vi "Homework-8 previous next Correct.vi"() -> ()   [LabVIEW 2016]
uses:
  <vilib>/Utility/file.llb/Read Delimited Spreadsheet (DBL).vi
panel:
  out "file name":string
  in  "stop":bool
  out "Waveform Graph":dbl[](graph)
  out "first row":dbl[](array[numeric])
  out "filenames":string[](array[string])
  out "folder names":string[](array[string])
  out "stripped path":path
  out "selected path":path
  out "File path":path
  in  "next":bool
  in  "previous":bool
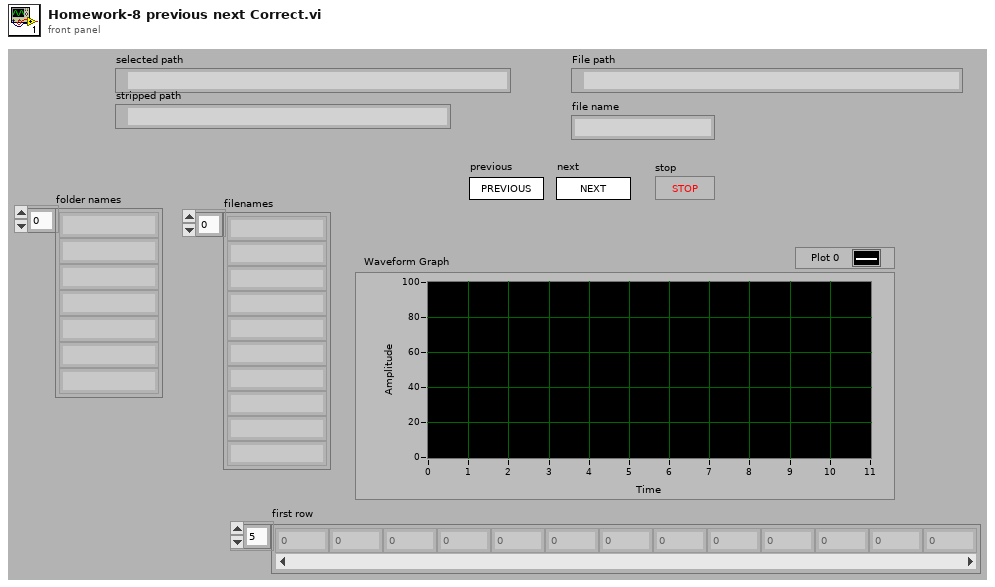
[diagram p1: front panel]
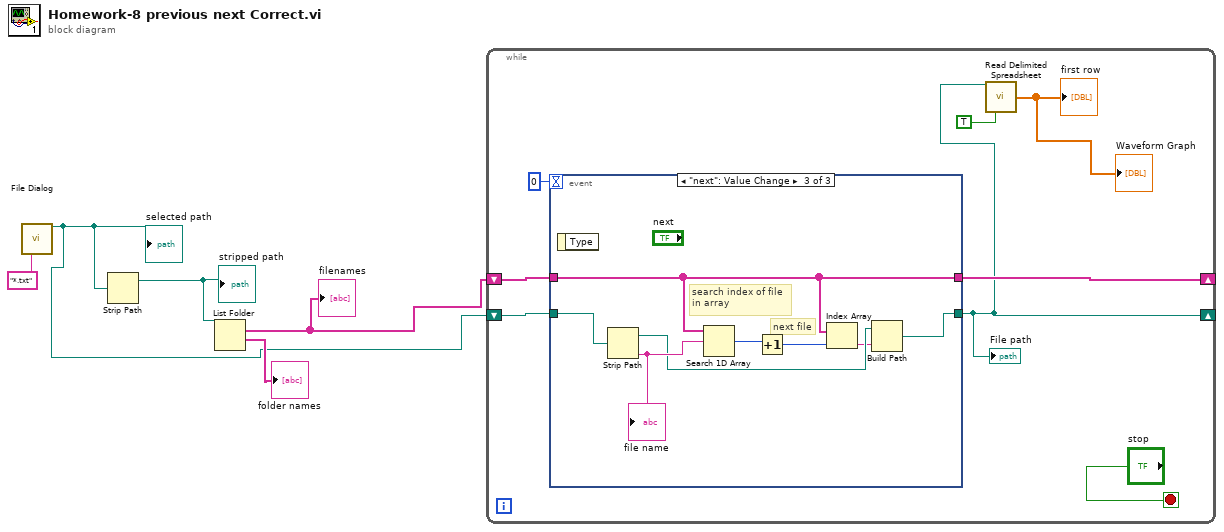
[diagram p0: block diagram]
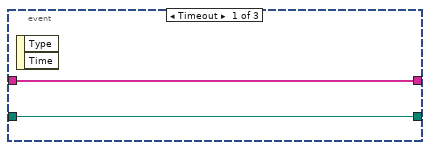
[diagram p2: hidden frame]
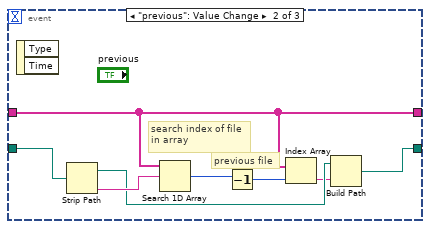
[diagram p3: hidden frame]
diagram:
  n1 = call "File Dialog"("pattern (all files)"="*.txt") -> ("selected path"=w1:path)  [unwired: 11 in, 3 out]
  "selected path" <- w1
  n2 = Strip Path(path=w1) -> (stripped path=w2:path)  [unwired: 1 out]
  "stripped path" <- w2
  n3 = List Folder(path=w2) -> (filenames=w3:string[], folder names=→"folder names":string[])  [unwired: 3 in, 2 out]
  "filenames" <- w3
  n4 = while {
    shift-right: [w13] -> _
    shift-left: w3 -> [w12]
    shift-right: [w8] -> _
    shift-left: w1 -> [w11]
    stop <- "stop" stop-if-true
    n5 = event shown="[2] \"next\": Value Change" {
      selector: _ -> [_ _ _]
      dyn-events: _ -> [_ _ _]
      timeout: 0 -> [_ _ _]
      tunnel: [w14 w16 w26] -> w8
      tunnel: [w15 w18 w24] -> w13
      tunnel: w12 -> [w15 w18 w24]
      tunnel: w11 -> [w14 w23 w25]
      event Timeout {
        n6 = event-data() -> ()  [unwired: 1 in, 2 out]
      }
      event "previous": Value Change {
        # "previous file"
        # "search index of file\nin array"
        n7 = event-data() -> ()  [unwired: 1 in, 2 out]
        n8 = Strip Path(path=w23) -> (stripped path=w20:path, name=w22:string)
        n9 = Search 1D Array(1D array=w18, element=w22) -> (index of element=w21:i32)  [unwired: 1 in]
        n10 = Decrement(x=w21) -> (x-1=w19:i32)
        n11 = Index Array(array=w18, index=w19) -> (element=w17:string)
        n12 = Build Path(base path=w20, name or relative path=w17) -> (appended path=w16:path)
      }
      event "next": Value Change {
        # "next file"
        # "search index of file\nin array"
        n13 = event-data() -> ()  [unwired: 1 in, 1 out]
        n14 = Strip Path(path=w25) -> (stripped path=w29:path, name=w31:string)
        "file name" <- w31
        n15 = Search 1D Array(1D array=w24, element=w31) -> (index of element=w30:i32)  [unwired: 1 in]
        n16 = Increment(x=w30) -> (x+1=w28:i32)
        n17 = Index Array(array=w24, index=w28) -> (element=w27:string)
        n18 = Build Path(base path=w29, name or relative path=w27) -> (appended path=w26:path)
      }
    }
    "File path" <- w8
    n19 = call-poly <vilib>:"Read Delimited Spreadsheet.vi"("file path (dialog if empty)"=w8, "transpose? (F)"=TRUE) -> ("first row"=→"first row" →"Waveform Graph":dbl[])  [unwired: 8 in, 5 out]
  }
